vi "Unpack For Grpc.vi"(8 "error in (no error)":errorcluster, 9 "Configuration / Resuls (Config)":enum16{"Configuration", "Results"}(ring), 10 "Any":T1, 11 "MeasurementPluginService in":refnum<class "Measurement Plugin Service.lvclass">) -> (0 "error out":errorcluster, 2 "Data Value":variant, 3 "MeasurementPluginService in":refnum<class "Measurement Plugin Service.lvclass">)   [LabVIEW 2020, in "MeasurementLink Measurement Server.lvlib" / "Measurement Plugin Service.lvclass"]
uses:
  Measurement Plugin Service.lvclass
  <vilib>/gRPC/LabVIEW gRPC Library/Shared/Any.ctl
  <vilib>/gRPC/LabVIEW gRPC Library/grpc-lvsupport-release.lvlib
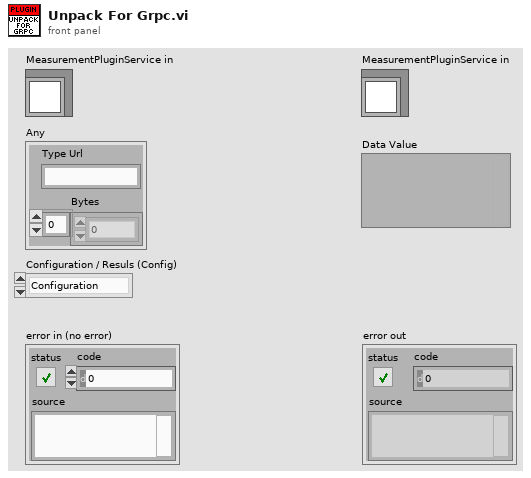
[diagram p1: front panel]
types:
  T1 = typedef "grpc-lvsupport-release.lvlib/Any.ctl" = cluster{"Type Url":string, "Bytes":u8[]}
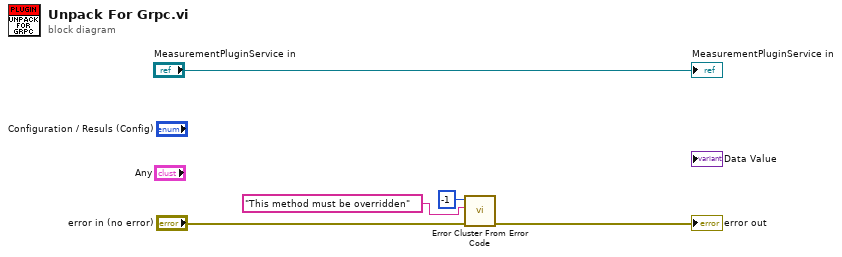
[diagram p0: block diagram]
diagram:
  n1 = call <vilib>:"Error Cluster From Error Code.vi"("error in (no error)"="error in (no error)", "error message (\"\")"="This method must be overridden" ("error message (\"\")"), "error code (0)"=-1) -> ("error out"=→"error out":errorcluster)  [unwired: 6 in]
  "MeasurementPluginService in" <- "MeasurementPluginService in"
